vi "Create HASH.vi"(11 "string":string) -> (3 "hash":i32)   [LabVIEW 2023]
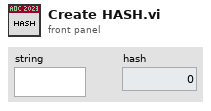
[diagram p1: front panel]
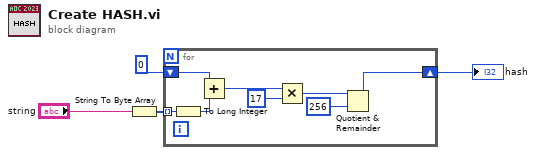
[diagram p0: block diagram]
diagram:
  n1 = String To Byte Array(string="string") -> (unsigned byte array=w1:u8[])
  n2 = for {
    tunnel: w1 -> [w7] mode=indexing
    shift-right: [w6] -> w4
    shift-left: 0 -> [w9]
    n3 = To Long Integer(number=w7) -> (32bit integer=w5:i32)
    n4 = Add(x=w9, y=w5) -> (x+y=w8:i32)
    n5 = Multiply(x=w8, y=17) -> (x*y=w11:i32)
    n6 = Quotient & Remainder(x=w11, y=256) -> (x-y*floor(x/y)=w6:i32)  [unwired: 1 out]
  }
  "hash" <- w4
